vi "cv4 visa.vi"() -> ()   [LabVIEW 2023]
panel:
  out "Array":string[](array[string])
  out "Array 2":string[][](array[string])
  out "transposed matrix":dbl[][](array[numeric]) format="%#_19g"
  out "Waveform Graph":dbl[][](graph)
  in  "stop":bool
  out "String":string
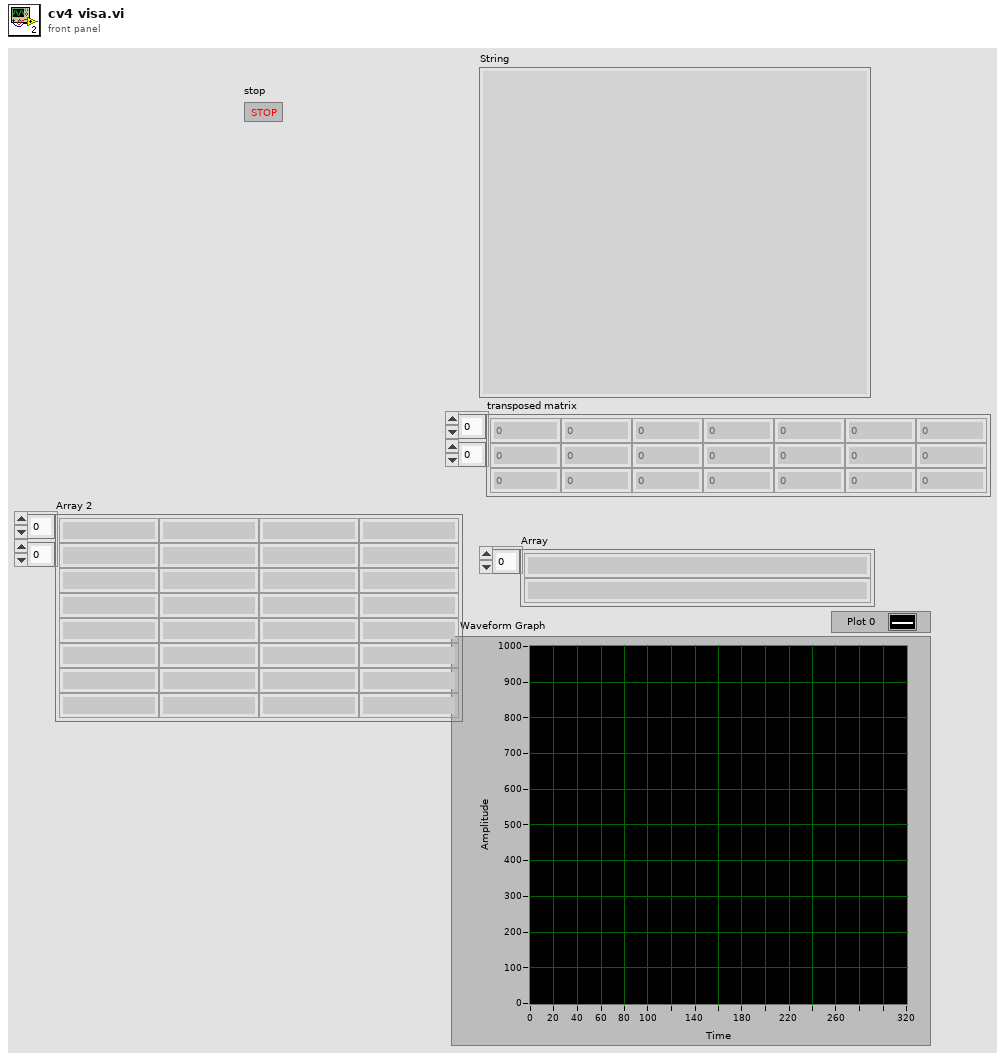
[diagram p1: front panel]
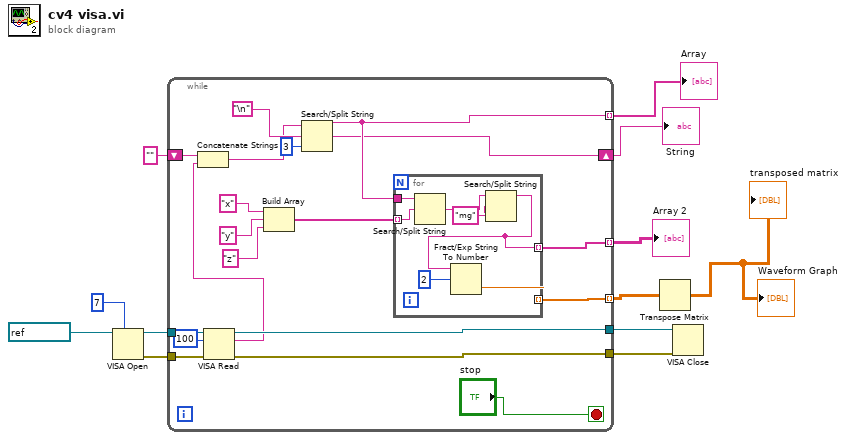
[diagram p0: block diagram]
diagram:
  n1 = VISA Open(timeout (0)=u32 7 ("VISA Open timeout (0)"), VISA resource name=refnum<visa-resource-name> "COM3") -> (VISA resource name=w10:refnum<visa-resource-name>, error out=w9:errorcluster)  [unwired: 3 in]
  n2 = while {
    tunnel: w10 -> [w31]
    tunnel: w9 -> [w30]
    tunnel: [w29] -> w8
    tunnel: [w28] -> w7
    shift-right: [w15] -> w2
    shift-left: "" -> [w27]
    tunnel: [w13] -> w5 mode=indexing
    tunnel: [w21] -> w3 mode=indexing
    tunnel: [w18] -> w1 mode=indexing
    stop <- "stop" stop-if-true
    n3 = VISA Read(VISA resource name=w31, byte count=u32 100, error in (no error)=w30) -> (VISA resource name out=w29:refnum<visa-resource-name>, read buffer=w19:string, error out=w28:errorcluster)  [unwired: 1 out]
    n4 = Concatenate Strings(w27, w19) -> (w16:string)
    n5 = Build Array("x" ("search string/char (-)"), "y" ("search string/char (-)"), "z" ("search string/char (-)")) -> (w24:string[])
    n6 = Search/Split String(string=w16, search string/char (-)="\n", offset (0)=3) -> (substring before match=w18:string, match + rest of string=w15:string)  [unwired: 1 out]
    n7 = for {
      tunnel: w24 -> [w38] mode=indexing
      tunnel: [w36] -> w13 mode=indexing
      tunnel: [w33] -> w21 mode=indexing
      tunnel: w18 -> [w32]
      n8 = Search/Split String(string=w32, search string/char (-)=w38) -> (match + rest of string=w35:string)  [unwired: 1 in, 2 out]
      n9 = Search/Split String(string=w35, search string/char (-)="mg") -> (substring before match=w33:string)  [unwired: 1 in, 2 out]
      n10 = Fract/Exp String To Number(string=w33, offset=2) -> (number=w36:dbl)  [unwired: 2 in, 1 out]
    }
  }
  "String" <- w2
  "Array 2" <- w3
  "Array" <- w1
  n11 = Transpose Matrix(1:w5) -> (0:→"Waveform Graph" →"transposed matrix":dbl[][])
  n12 = VISA Close(VISA resource name=w8, error in (no error)=w7) -> ()  [unwired: 1 out]
